vi "Get URI.vi"(11 "IUnregister in":refnum<class "IUnregister.lvclass">) -> (2 "URL":string, 3 "IUnregister out":refnum<class "IUnregister.lvclass">)   [LabVIEW 2020, in "wamplv.lvlib" / "IUnregister.lvclass"]
uses:
  IUnregister.lvclass
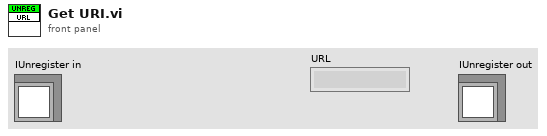
[diagram p1: front panel]
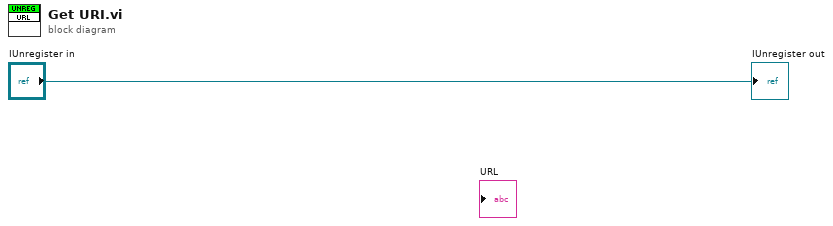
[diagram p0: block diagram]
diagram:
  "IUnregister out" <- "IUnregister in"
